vi "Less Than.vi"(1 "y":refnum<class "People By Month Wrapper.lvclass">, 2 "x":refnum<class "People By Month Wrapper.lvclass">) -> (0 "less than?":bool)   [LabVIEW 2023, in "People By Month Wrapper.lvclass"]
doc: "Returns TRUE if the value of <b>x</b> is less than the value of <b>y</b>."
uses:
  People By Month Wrapper.lvclass
  People By Month Wrapper.lvclass/People By Month Wrapper.ctl
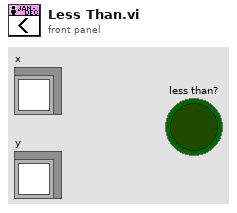
[diagram p1: front panel]
types:
  T1 = typedef "Person Information.ctl" = cluster{"ID":u32, "Family Name":string, "Given Name":string, "Birth Date":timestamp}
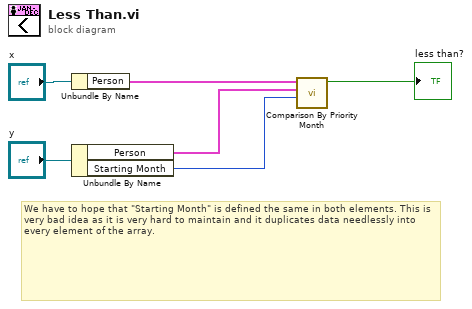
[diagram p0: block diagram]
diagram:
  # "We have to hope that \"Starting Month\" is defined the same in both elements. This is very bad idea as it is very hard to maintain and it duplicates data needlessly into every element of the array."
  n1 = Unbundle By Name("x") -> ("Person"=w4:T1)
  n2 = Unbundle By Name("y") -> ("Person"=w3:T1, "Starting Month"=w1:u32)
  n3 = call "Comparison By Priority Month.vi"("Starting Month"=w1, "Person B"=w3, "Person A"=w4) -> ("Swap?"=→"less than?":bool)  [unwired: 8 in]
